vi "PID-Profile.vi"(0 "Setpoint":dbl, 1 "Process variable":dbl, 3 "Trapezoidal Deceleration":bool, 4 "Slew Rate Limit":bool, 5 "Distance Range (+/-)":dbl=2.0, 6 "Upper Limit":dbl=1.0, 7 "Lower limit":dbl=-1.0, 8 "FeedFoward":dbl, 9 "Max Acceleration (units/sec^2)":dbl, 10 "Kp":dbl, 11 "Max Velocity (units/sec)":dbl, 12 "Kd":dbl) -> (14 "Output":dbl, 19 "At Goal":bool)   [LabVIEW 2020]
uses:
  <vilib>/Rock Robotics/WPI/ThirdParty/JAS_Junk/TrajLib/Trajectory_Library.lvlib
panel:
  # "Inputs"
  # "Constants"
  # "Outputs"
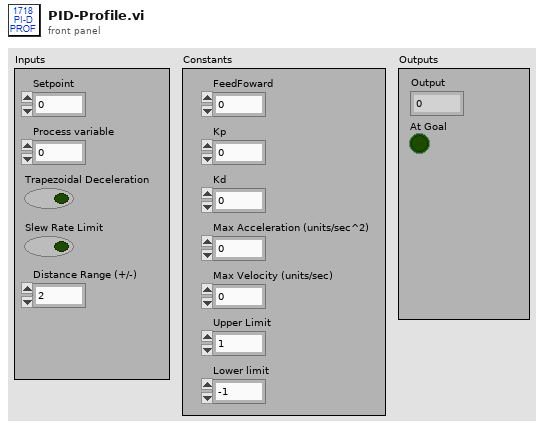
[diagram p1: front panel]
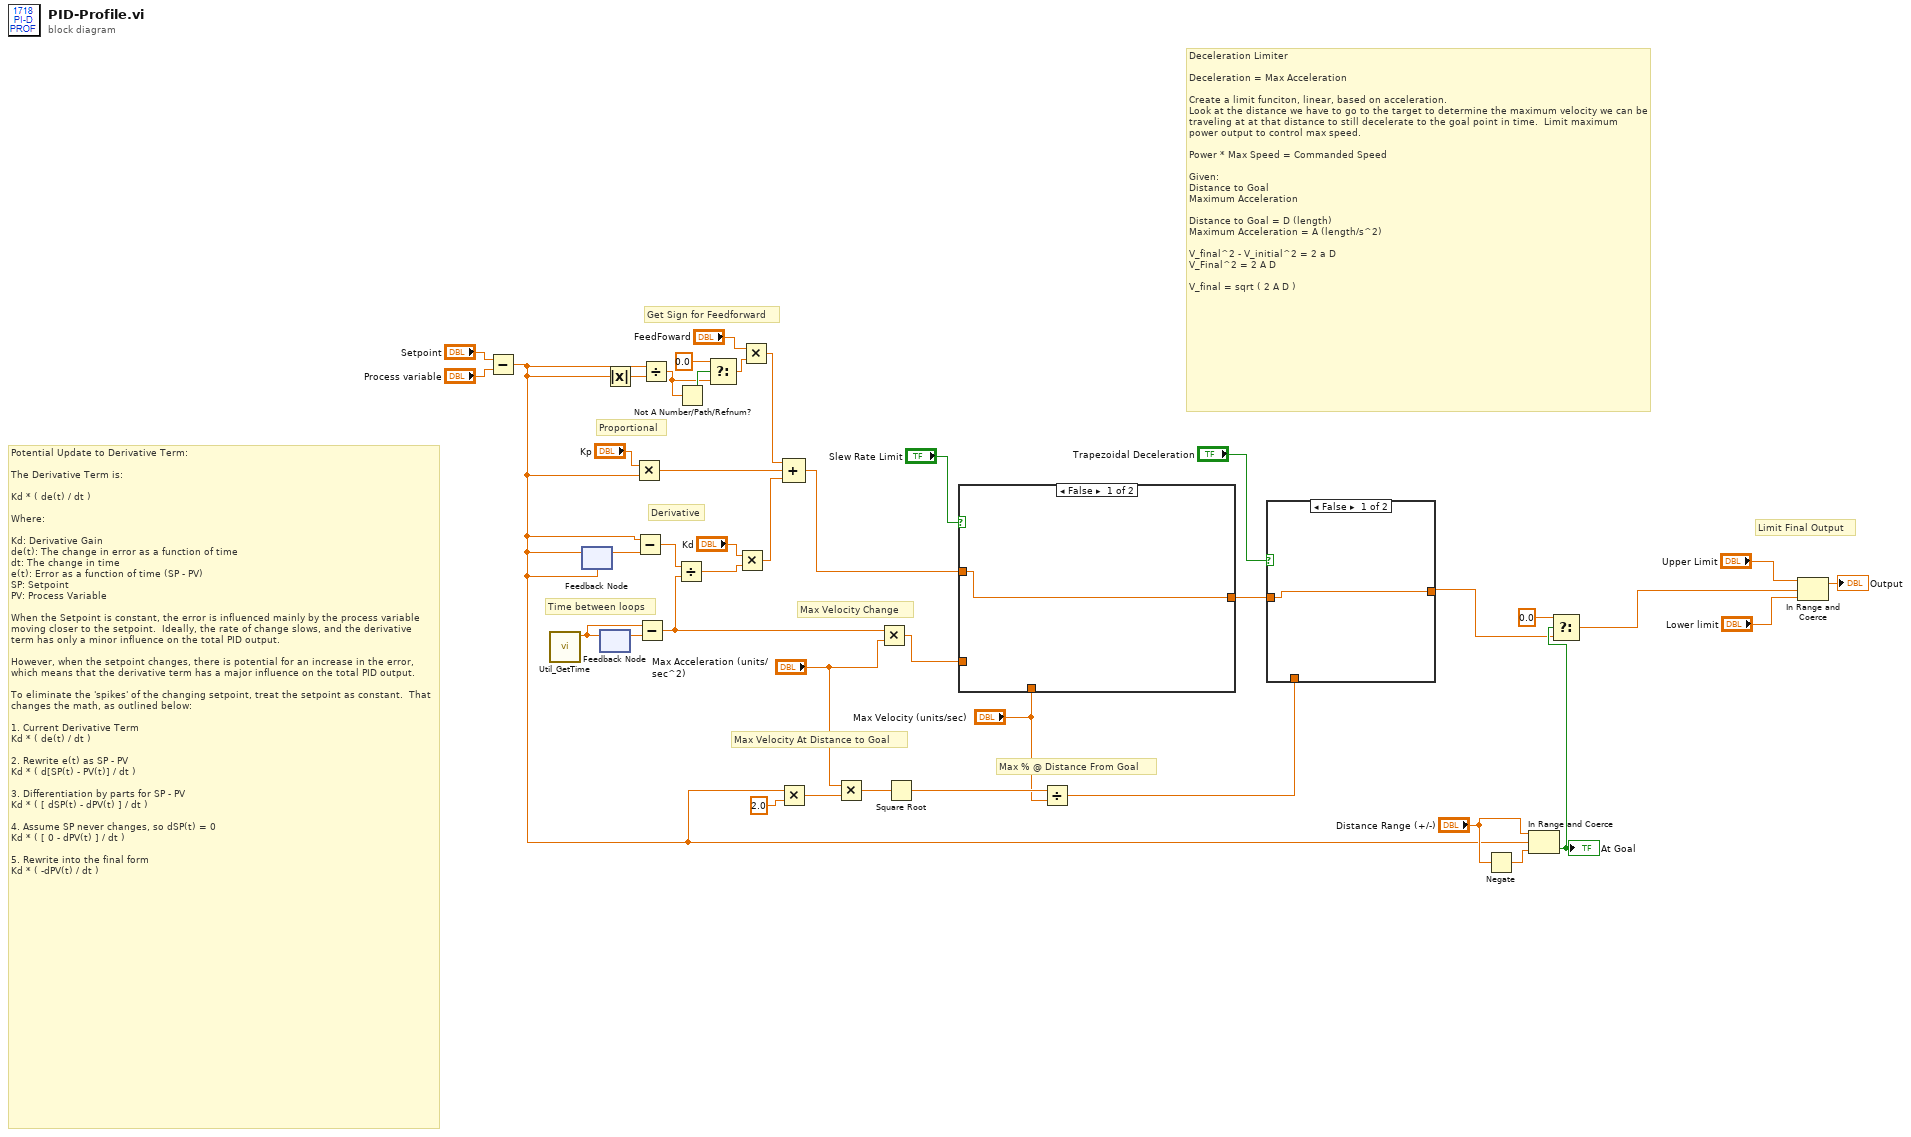
[diagram p0: block diagram]
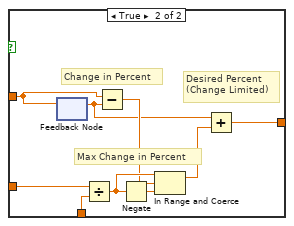
[diagram p2: hidden frame]
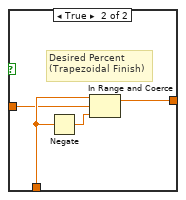
[diagram p3: hidden frame]
diagram:
  # "Potential Update to Derivative Term:\n\nThe Derivative Term is:\n\nKd * ( de(t) / dt )\n\nWhere:\n\nKd: Derivative Gain\nde(t): The change in error as a function of time\ndt: The change in time\ne(t): Error as a function of time (SP - PV)\nSP: Setpoint\nPV: Process Variable\n\nWhen the Setpoint is constant, the error is influenced mainly by the process variable moving closer to the setpoint.  Ideally, the rate of change slows, and the derivative term has only a minor influence on the total PID output.\n\nHowever, when the setpoint changes, there is potential for an increase in the error, which means that the derivative term has a major influence on the total PID output.\n\nTo eliminate the 'spikes' of the changing setpoint, treat the setpoint as constant.  That changes the math, as outlined below:\n\n1. Current Derivative Term\nKd * ( de(t) / dt )\n\n2. Rewrite e(t) as SP - PV\nKd * ( d[SP(t) - PV(t)] / dt )\n\n3. Differentiation by parts for SP - PV\nKd * ( [ dSP(t) - dPV(t) ] / dt )\n\n4. Assume SP never changes, so dSP(t) = 0\nKd * ( [ 0 - dPV(t) ] / dt )\n\n5. Rewrite into the final form\nKd * ( -dPV(t) / dt )"
  # "Max % @ Distance From Goal"
  # "Max Velocity At Distance to Goal"
  # "Deceleration Limiter\n\nDeceleration = Max Acceleration\n\nCreate a limit funciton, linear, based on acceleration.\nLook at the distance we have to go to the target to determine the maximum velocity we can be traveling at at that distance to still decelerate to the goal point in time.  Limit maximum power output to control max speed.\n\nPower * Max Speed = Commanded Speed\n\nGiven:\nDistance to Goal\nMaximum Acceleration\n\nDistance to Goal = D (length)\nMaximum Acceleration = A (length/s^2)\n\nV_final^2 - V_initial^2 = 2 a D\nV_Final^2 = 2 A D\n\nV_final = sqrt ( 2 A D )"
  # "Max Velocity Change"
  # "Limit Final Output"
  # "Derivative"
  # "Proportional"
  # "Time between loops"
  # "Get Sign for Feedforward"
  n1 = Subtract(x="Setpoint", y="Process variable") -> (x-y=w11:dbl)
  n2 = call <vilib>:"Util_GetTime.vi"() -> ("FPGA_Time_Seconds"=w27:dbl)  [unwired: 10 in, 1 out]
  n3 = feedback #1(w11) -> (w35:dbl)
  n4 = feedback-in #1(w11) -> ()
  n5 = feedback #2() -> (w37:dbl)  [unwired: 1 in]
  n6 = feedback-in #2(w27) -> ()
  n7 = Absolute Value(x=w11) -> (abs(x)=w39:dbl)
  n8 = Multiply(x="Kp", y=w11) -> (x*y=w30:dbl)
  n9 = Subtract(x=w11, y=w35) -> (x-y=w34:dbl)
  n10 = Subtract(x=w27, y=w37) -> (x-y=w26:dbl)
  n11 = Divide(x=w11, y=w39) -> (x/y=w6:dbl)
  n12 = Divide(x=w34, y=w26) -> (x/y=w33:dbl)
  n13 = Not A Number/Path/Refnum?(number/path/refnum=w6) -> (NaN/Path/Refnum?=w8:bool)
  n14 = Select(t=0.0, s=w8, f=w6) -> (s? t:f=w5:dbl)
  n15 = Multiply(x="Kd", y=w33) -> (x*y=w29:dbl)
  n16 = Multiply(x="FeedFoward", y=w5) -> (x*y=w31:dbl)
  n17 = Multiply(x=w11, y=2.0) -> (x*y=w21:dbl)
  n18 = Compound Arithmetic op=ADD(w31, w30, w29) -> (w25:dbl)
  n19 = Multiply(x="Max Acceleration (units/sec^2)", y=w21) -> (x*y=w20:dbl)
  n20 = Multiply(x=w26, y="Max Acceleration (units/sec^2)") -> (x*y=w24:dbl)
  n21 = Square Root(x=w20) -> (sqrt(x)=w19:dbl)
  n22 = case shown="False" "Slew Rate Limit" {
    tunnel: w25 -> [w42 w51]
    tunnel: w24 -> [_ w50]
    tunnel: "Max Velocity (units/sec)" -> [_ w44]
    tunnel: [w42 w43] -> w16
    frame False {
    }
    frame True {
      # "Desired Percent\n(Change Limited)"
      # "Max Change in Percent"
      # "Change in Percent"
      n23 = feedback #3() -> (w45:dbl)  [unwired: 1 in]
      n24 = feedback-in #3(w51) -> ()
      n25 = Divide(x=w50, y=w44) -> (x/y=w48:dbl)
      n26 = Subtract(x=w51, y=w45) -> (x-y=w47:dbl)
      n27 = Negate(x=w48) -> (-x=w49:dbl)
      n28 = In Range and Coerce(upper limit=w48, x=w47, lower limit=w49) -> (coerced(x)=w46:dbl)  [unwired: 1 out]
      n29 = Add(x=w45, y=w46) -> (x+y=w43:dbl)
    }
  }
  n30 = Divide(x=w19, y="Max Velocity (units/sec)") -> (x/y=w17:dbl)
  n31 = case shown="False" "Trapezoidal Deceleration" {
    tunnel: w17 -> [_ w55]
    tunnel: [w52 w54] -> w2
    tunnel: w16 -> [w52 w53]
    frame False {
    }
    frame True {
      # "Desired Percent\n(Trapezoidal Finish)"
      n32 = Negate(x=w55) -> (-x=w56:dbl)
      n33 = In Range and Coerce(upper limit=w55, x=w53, lower limit=w56) -> (coerced(x)=w54:dbl)  [unwired: 1 out]
    }
  }
  n34 = Negate(x="Distance Range (+/-)") -> (-x=w13:dbl)
  n35 = In Range and Coerce(upper limit="Distance Range (+/-)", x=w11, lower limit=w13) -> (In Range?=w4:bool)  [unwired: 1 out]
  "At Goal" <- w4
  n36 = Select(t=0.0, s=w4, f=w2) -> (s? t:f=w1:dbl)
  n37 = In Range and Coerce(upper limit="Upper Limit", x=w1, lower limit="Lower limit") -> (coerced(x)=→"Output":dbl)  [unwired: 1 out]
